vi "Write Sweep Element.vi"(6 "loop index":i32, 8 "error in (no error)":errorcluster, 9 "value":variant, 10 "key":string, 11 "Control Experiment in":refnum<class "Control Experiment SM.lvclass">) -> (0 "error out":errorcluster, 3 "Control Experiment out":refnum<class "Control Experiment SM.lvclass">)   [LabVIEW 2016, in "Control Experiment SM.lvclass"]
uses:
  Control Experiment SM.lvclass
  Control Experiment SM.lvclass/Control Experiment SM.ctl
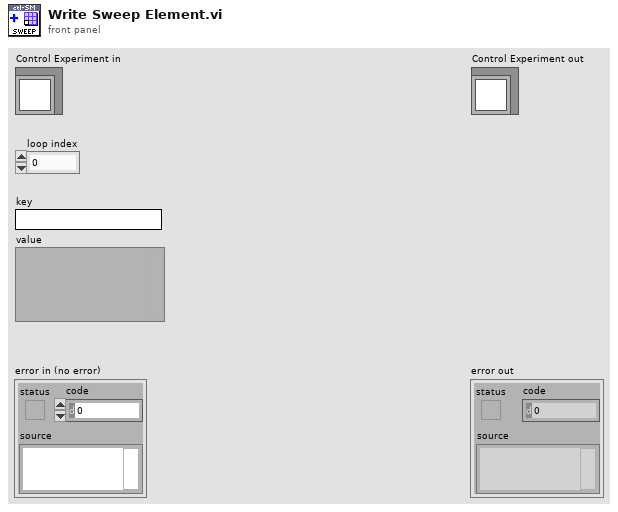
[diagram p1: front panel]
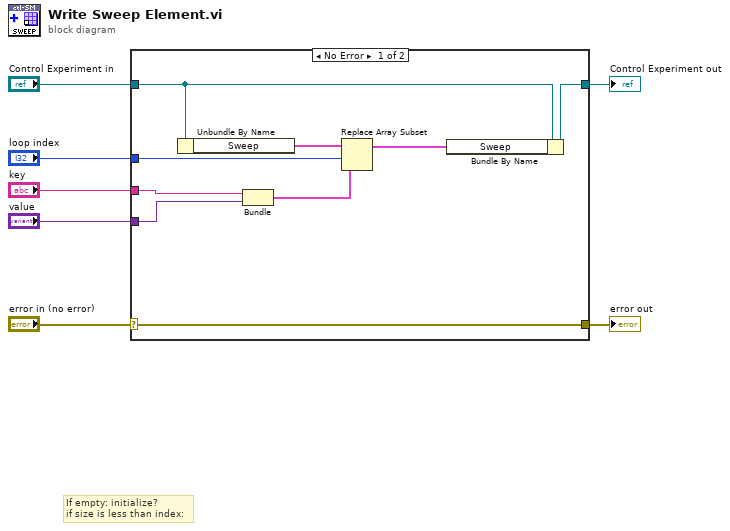
[diagram p0: block diagram]
diagram:
  # "If empty: initialize?\nif size is less than index:"
  n1 = case shown="No Error" "error in (no error)" {
    selector: "error in (no error)" -> [w16 w17]
    tunnel: [w16 w17] -> w6
    tunnel: [w15 w18] -> w4
    tunnel: "Control Experiment in" -> [w12 w18]
    tunnel: "loop index" -> [w10 _]
    tunnel: "key" -> [w14 _]
    tunnel: "value" -> [w13 _]
    frame No Error {
      n2 = Unbundle By Name(w12) -> ("Sweep"=w9:cluster{"key":string, "value":variant}[])
      n3 = Bundle("key"=w14, "value"=w13) -> (w11:cluster{"key":string, "value":variant})  [unwired: 1 in]
      n4 = Replace Array Subset(array=w9, new element=w11, index=w10) -> (w8:cluster{"key":string, "value":variant}[])
      n5 = Bundle By Name(cluster=w12, "Sweep"=w8) -> (w15:refnum<class "Control Experiment SM.lvclass">)
    }
    frame Error {
    }
  }
  "error out" <- w6
  "Control Experiment out" <- w4
